vi "RS-xxx to GPIB ConvBox Factory.vi"(8 "error in (no error)":errorcluster, 10 "RS-xxx to GPIB ConvBox settings":T1) -> (0 "error out":errorcluster, 3 "protocol out":refnum<class "Protocol Parent.lvclass">)   [LabVIEW 2023, in "Protocols.lvlib" / "RS-xxx to GPIB ConvBox.lvclass"]
doc: "Instantiates a new RS-xxx to GPIB ConvBox Protocol object using the provided RS-xxx to GPIB ConvBox settings."
uses:
  RS-xxx to GPIB ConvBox.lvclass
  Protocol Parent/Protocol Parent.lvclass
  RS-xxx to GPIB ConvBox Settings.ctl
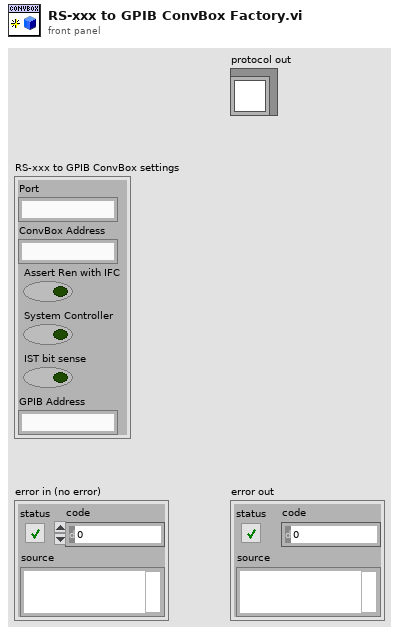
[diagram p1: front panel]
types:
  T1 = typedef "Protocols.lvlib/RS-xxx to GPIB ConvBox.lvclass/RS-xxx to GPIB ConvBox Settings.ctl" = cluster{"Port":string, "ConvBox Address":string, "Assert Ren with IFC":bool, "System Controller":bool, "IST bit sense":bool, "GPIB Address":string}
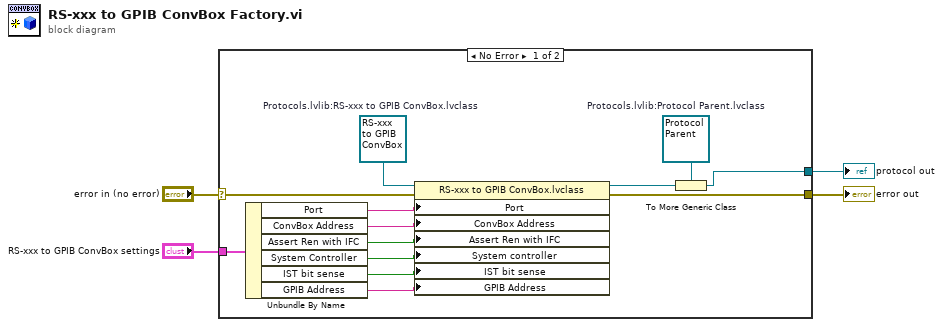
[diagram p0: block diagram]
diagram:
  n1 = case shown="No Error" "error in (no error)" {
    selector: "error in (no error)" -> [w9 w18]
    tunnel: "RS-xxx to GPIB ConvBox settings" -> [w17 _]
    tunnel: [w5 _] -> w1
    tunnel: [w15 w18] -> w3
    frame No Error {
      w6 = refnum<class "Protocol Parent.lvclass"> refnum  # Protocols.lvlib:Protocol Parent.lvclass
      w16 = refnum<class "RS-xxx to GPIB ConvBox.lvclass"> refnum  # Protocols.lvlib:RS-xxx to GPIB ConvBox.lvclass
      n2 = Unbundle By Name(w17) -> ("Port"=w8:string, "ConvBox Address"=w14:string, "Assert Ren with IFC"=w13:bool, "System Controller"=w12:bool, "IST bit sense"=w11:bool, "GPIB Address"=w10:string)
      n3 = property class="RS-xxx to GPIB ConvBox.lvclass"(reference=w16, error in=w9, "Port"=w8, "ConvBox Address"=w14, "Assert Ren with IFC"=w13, "System controller"=w12, "IST bit sense"=w11, "GPIB Address"=w10) -> (reference out=w7:refnum<class "RS-xxx to GPIB ConvBox.lvclass">, error out=w15:errorcluster)
      n4 = To More Generic Class(target class=w6, reference=w7) -> (generic class reference=w5:refnum<class "Protocol Parent.lvclass">)
    }
    frame Error {
    }
  }
  "error out" <- w3
  "protocol out" <- w1
